vi "Get Data Type Name.vi"(11 "LimitType in":refnum<class "Numeric Limit.lvclass">) -> (3 "Data Type Name":string="Default Data Type")   [LabVIEW 2017, in "Numeric Limit.lvclass"]
uses:
  Numeric Limit.lvclass
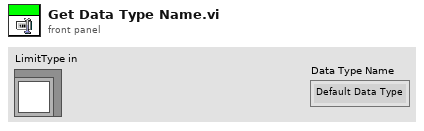
[diagram p1: front panel]
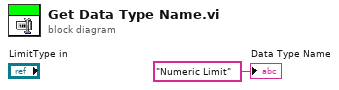
[diagram p0: block diagram]
diagram:
  "Data Type Name" <- "Numeric Limit" ("Data Type Name")
